vi "defineNamespace.vi"(8 "error in (no error)":errorcluster, 10 "Name":string, 11 "Test Runner in":refnum<class "Test Runner.lvclass">) -> (0 "error out":errorcluster, 2 "Namespace":string, 3 "Test Runner out":refnum<class "Test Runner.lvclass">)   [LabVIEW 2013, in "Caraya.lvlib" / "Test Runner.lvclass"]
uses:
  Test Runner.lvclass
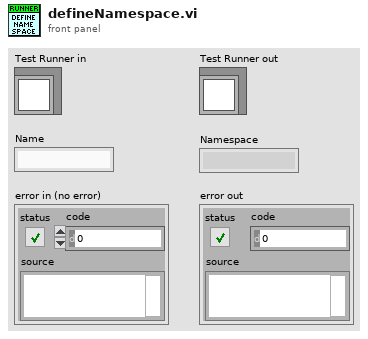
[diagram p1: front panel]
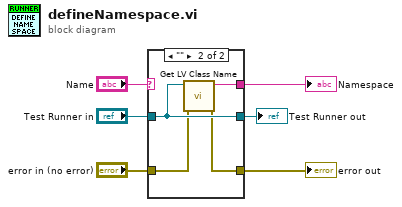
[diagram p0: block diagram]
diagram:
  n1 = case shown="\"\"" "Name" {
    selector: "Name" -> [w9 _]
    tunnel: [w9 w12] -> w4
    tunnel: "Test Runner in" -> [w8 w13]
    tunnel: [w8 w13] -> w3
    tunnel: "error in (no error)" -> [w7 w11]
    tunnel: [w7 w10] -> w6
    frame Default {
    }
    frame "" {
      n2 = call <vilib>:"Get LV Class Name.vi"("error in (no error)"=w11, "object"=w13) -> ("error out"=w10:errorcluster, "class name"=w12:string)  [unwired: 8 in]
    }
  }
  "error out" <- w6
  "Namespace" <- w4
  "Test Runner out" <- w3
